vi "ManualGantryControl.vi"(7 "MaxGantryIncrement":dbl, 10 "PrevGantrySetpoint":dbl, 11 "JoystickAxis":dbl[](array[numeric])) -> (2 "NewGantrySetpoint":dbl)   [LabVIEW 2014]
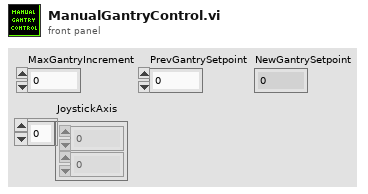
[diagram p1: front panel]
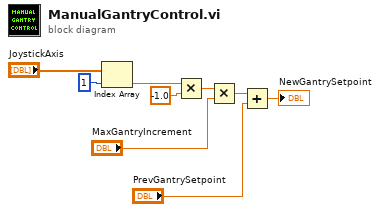
[diagram p0: block diagram]
diagram:
  n1 = Index Array(array="JoystickAxis", index=1) -> (element=w6:dbl)
  n2 = Multiply(x=w6, y=-1.0) -> (x*y=w5:dbl)
  n3 = Multiply(x=w5, y="MaxGantryIncrement") -> (x*y=w3:dbl)
  n4 = Add(x=w3, y="PrevGantrySetpoint") -> (x+y=→"NewGantrySetpoint":dbl)
